vi "serial.vi"() -> ()   [LabVIEW 2021]
uses:
  <vilib>/Instr/_visa.llb/VISA Configure Serial Port (Instr).vi
panel:
  in  "Puerto de Comunicacion":refnum<visa-resource-name>
  in  "stop":bool
  in  "Interruptores":bool[](array[boolean])
  out "LEDS":bool[](array[boolean])
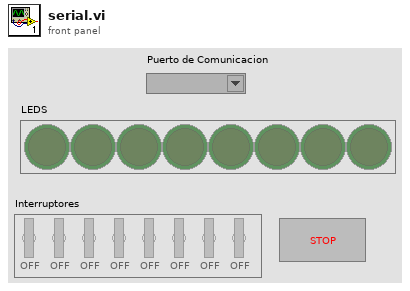
[diagram p1: front panel]
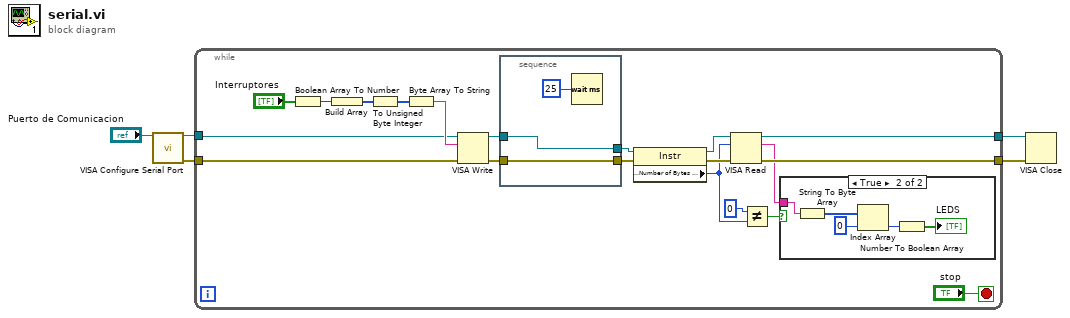
[diagram p0: block diagram]
diagram:
  n1 = call-poly "VISA Configure Serial Port"("VISA resource name"="Puerto de Comunicacion") -> ("VISA resource name out"=w4:refnum<visa-resource-name>, "error out"=w3:errorcluster)  [unwired: 8 in, 5 out]
  n2 = while {
    tunnel: w4 -> [w14]
    tunnel: w3 -> [w13]
    tunnel: [w12] -> w2
    tunnel: [w11] -> w1
    stop <- "stop" stop-if-true
    n3 = Boolean Array To Number(Boolean array="Interruptores") -> (number=w18:u32)
    n4 = Build Array(w18) -> (w16:u32[])
    n5 = To Unsigned Byte Integer(number=w16) -> (unsigned 8bit integer=w15:u8[])
    n6 = Byte Array To String(unsigned byte array=w15) -> (string=w17:string)
    n7 = VISA Write(VISA resource name=w14, write buffer=w17, error in (no error)=w13) -> (VISA resource name out=w23:refnum<visa-resource-name>, error out=w25:errorcluster)  [unwired: 1 out]
    n8 = stacked-sequence {
      tunnel: w25 -> [w33]
      tunnel: [w33] -> w24
      tunnel: w23 -> [w32]
      tunnel: [w32] -> w22
      frame #0 {
        n9 = Wait (ms)(milliseconds to wait=u32 25) -> ()  [unwired: 1 out]
      }
    }
    n10 = property class="Instr"(reference=w22, error in=w24) -> (reference out=w21:refnum<visa-resource-name>, error out=w20:errorcluster, "Serial Settings:Number of Bytes at Serial Port"=w10:u32)
    n11 = VISA Read(VISA resource name=w21, byte count=w10, error in (no error)=w20) -> (VISA resource name out=w12:refnum<visa-resource-name>, read buffer=w7:string, error out=w11:errorcluster)  [unwired: 1 out]
    n12 = Not Equal?(x=u32 0, y=w10) -> (x != y?=w8:bool)
    n13 = case shown="True" w8 {
      tunnel: w7 -> [_ w28]
      frame False {
      }
      frame True {
        n14 = String To Byte Array(string=w28) -> (unsigned byte array=w30:u8[])
        n15 = Index Array(array=w30, index=0) -> (element=w27:u8)
        n16 = Number To Boolean Array(number=w27) -> (Boolean array=→"LEDS":bool[])
      }
    }
  }
  n17 = VISA Close(VISA resource name=w2, error in (no error)=w1) -> ()  [unwired: 1 out]
